vi "3.1-Where.vi"() -> (1 "Heartbeat":bool, 2 "Consolidated Where Data":T1 {"Current GPS Data"."Longitude (dd.mmmmmm)" format="%#.6g"; "Current GPS Data"."Lattitude (dd.mmmmmm)" format="%#.6g"})   [LabVIEW 2010]
uses:
  4-High Neurons/Current GPS Data.ctl
  3.1-Where/_typedefs/ConsolidatedWhereData.ctl
  3.1-Where/3.1.1-VectorNav/3.1.1-VectorNav Data.ctl
  3.0-Global.vi
panel:
  out "Current GPS Data":T2 {"Longitude (dd.mmmmmm)" format="%#.6g"; "Lattitude (dd.mmmmmm)" format="%#.6g"}
  # "GPS"
  # "VectorNav"
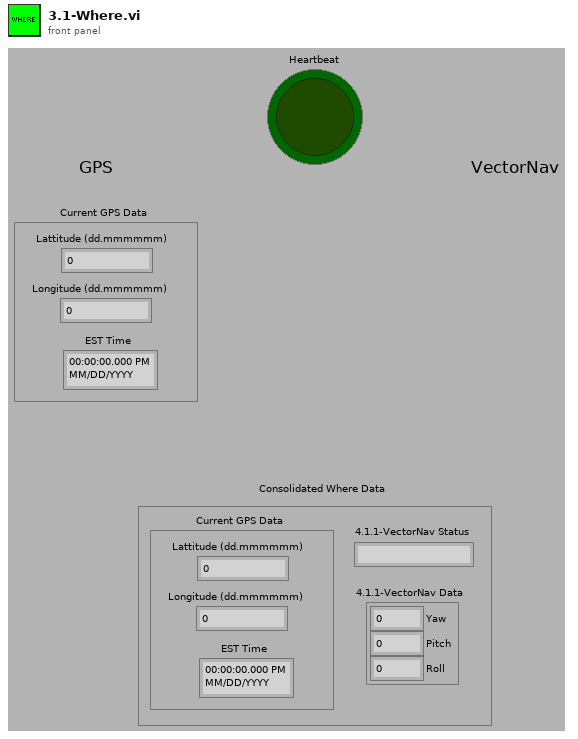
[diagram p1: front panel]
types:
  T1 = typedef "ConsolidatedWhereData.ctl" = cluster{"Current GPS Data":T2, "4.1.1-VectorNav Data":T3, "4.1.1-VectorNav Status":string}
  T2 = typedef "Current GPS Data.ctl" = cluster{"Lattitude (dd.mmmmmm)":dbl, "Longitude (dd.mmmmmm)":dbl, "EST Time":timestamp}
  T3 = typedef "3.1.1-VectorNav Data.ctl" = cluster{"Yaw":dbl, "Pitch":dbl, "Roll":dbl}
  T4 = typedef "2-FPGA VI Typedef.ctl" = refnum<k20>
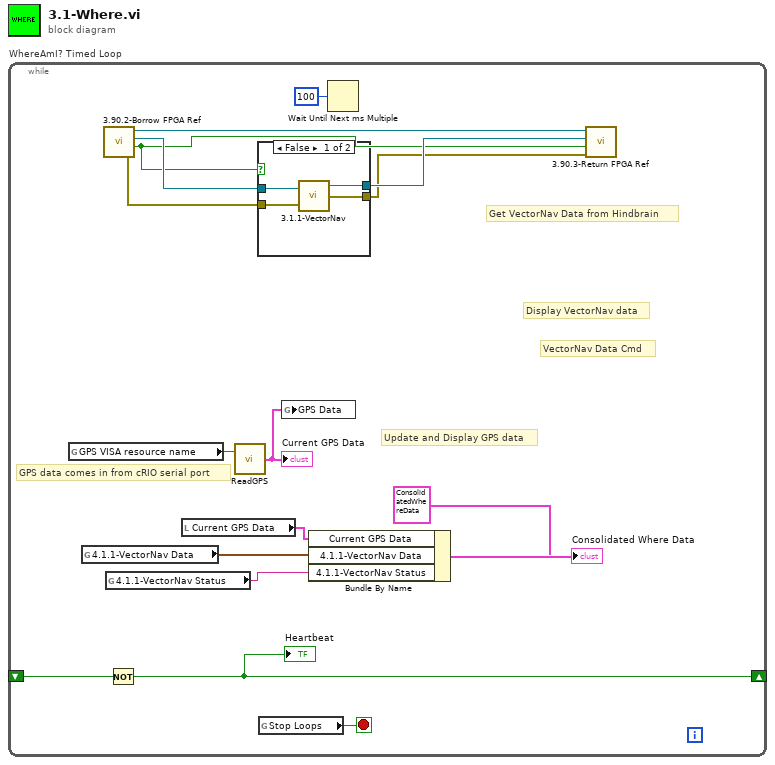
[diagram p0: block diagram]
diagram:
  n1 = while "WhereAmI? Timed Loop" {
    shift-right: [w16] -> _
    shift-left: _ -> [w17]
    stop <- w15 stop-if-true
    # "GPS data comes in from cRIO serial port"
    # "Update and Display GPS data"
    # "VectorNav Data Cmd"
    # "Display VectorNav data"
    # "Get VectorNav Data from Hindbrain"
    n2 = global read "3.0-Global.vi" "GPS VISA resource name"() -> (w1:refnum<visa-resource-name>)
    n3 = global read "3.0-Global.vi" "4.1.1-VectorNav Data"() -> (w4:T3)
    n4 = call "3.90.2-Borrow FPGA Ref.vi"() -> ("error out"=w11:errorcluster, "Failed to Obtain Ref"=w8:bool, "element"=w12:T4, "FPGA Ref"=w13:refnum<queue>)  [unwired: 4 in]
    n5 = global read "3.0-Global.vi" "4.1.1-VectorNav Status"() -> (w3:string)
    n6 = Not(x=w17) -> (.not. x?=w16:bool)
    "Heartbeat" <- w16
    n7 = local read "Current GPS Data"() -> (w5:T2)
    n8 = call "ReadGPS.vi"("VISA resource name"=w1) -> ("Current GPS Data"=w2:T2)  [unwired: 1 in]
    "Current GPS Data" <- w2
    n9 = case shown="False" w8 {
      tunnel: [w21 w22] -> w9
      tunnel: [w20 w23] -> w10
      tunnel: w12 -> [w19 w23]
      tunnel: w11 -> [w18 w22]
      frame False {
        n10 = call "3.1.1-VectorNav.vi"("error in"=w18, "FPGA Ref In"=w19) -> ("error out"=w21:errorcluster, "FPGA Ref Out"=w20:T4)  [unwired: 1 out]
      }
      frame True {
      }
    }
    n11 = global read "3.0-Global.vi" "Stop Loops"() -> (w15:bool)
    n12 = global write "3.0-Global.vi" "GPS Data"(w2) -> ()
    n13 = Bundle By Name(cluster=T1 {"Current GPS Data"={"Lattitude (dd.mmmmmm)"=0.0, "Longitude (dd.mmmmmm)"=0.0, "EST Time"=timestamp(0 s since 1904-01-01)}, "4.1.1-VectorNav Data"={"Yaw"=0.0, "Pitch"=0.0, "Roll"=0.0}, "4.1.1-VectorNav Status"=""} ("Consolidated Where Data 2"), "Current GPS Data"=w5, "4.1.1-VectorNav Data"=w4, "4.1.1-VectorNav Status"=w3) -> (→"Consolidated Where Data":T1)
    n14 = Wait Until Next ms Multiple(millisecond multiple=u32 100) -> ()  [unwired: 1 out]
    n15 = call "3.90.3-Return FPGA Ref.vi"("error in"=w9, "Failed to Obtain Ref"=w8, "element"=w10, "FPGA Ref"=w13) -> ()  [unwired: 1 out]
  }
